vi "DSF.Engine.Execution.BuilderManager.Create.vi"(8 "error in (no error)":errorcluster, 10 "number of builders":i32, 11 "Framework Cache":refnum<class "DSF.Engine.Memory.Cache.Framework.lvclass">) -> (0 "error out":errorcluster, 3 "Builder Manager out":refnum<class "DSF.Engine.Execution.BuilderManager.lvclass">)   [LabVIEW 2016, in "DSF.Engine.lvlib" / "DSF.Engine.Execution.BuilderManager.lvclass"]
uses:
  DSF.Engine.Execution.BuilderManager.lvclass
  Cache/DSF.Engine.Memory.Cache.Framework.lvclass
  Builder/DSF.Engine.Execution.Builder.lvclass/DSF.Engine.Execution.Builder.ctl
  DSF.Engine.Execution.BuilderManager.lvclass/DSF.Engine.Execution.BuilderManager.ctl
  Builder/DSF.Engine.Execution.Builder.Set FIFOs.vi
  Builder/DSF.Engine.Execution.Builder.Set Status Pointers.vi
  Submodules/Memory/Source/Classes/Standard Types/Memory.Pointer.U32.New.vi
  Builder/DSF.Engine.Execution.Builder.Set Framework Cache.vi
  Submodules/Memory/Source/Classes/Standard Types/Memory.Pointer.U32.lvclass
  C:/Git/Sourcetree/DSF/Source/Submodules/Memory/Source/Classes/Internal/Memory.Pointer.Internal.lvclass
  Submodules/Memory/Source/Classes/Internal/Memory.Pointer.Internal.Allocate.vi
  Builder/DSF.Engine.Execution.Builder.lvclass
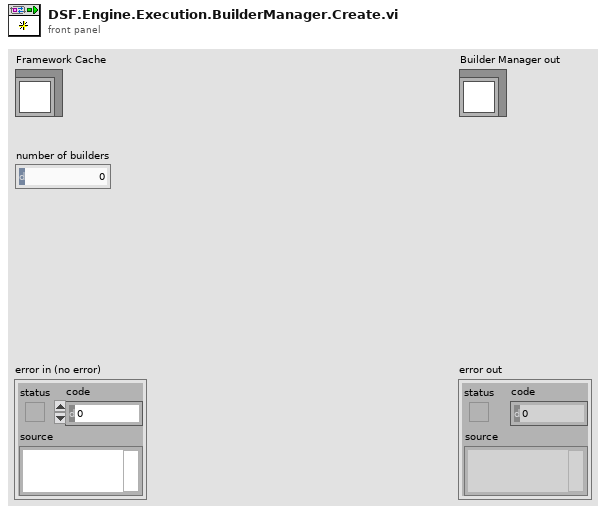
[diagram p1: front panel]
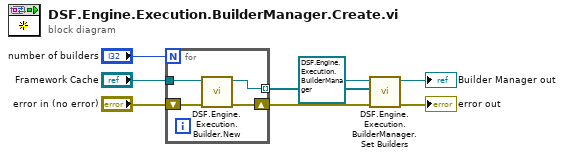
[diagram p0: block diagram]
diagram:
  n1 = for {
    N: "number of builders" -> [_]
    shift-right: [w11] -> w5
    shift-left: "error in (no error)" -> [w12]
    tunnel: [w10] -> w4 mode=indexing
    tunnel: "Framework Cache" -> [w9]
    n2 = call "DSF.Engine.Execution.Builder.New.vi"("error in (no error)"=w12, "Framework Cache"=w9) -> ("error out"=w11:errorcluster, "Builder"=w10:refnum<class "DSF.Engine.Execution.Builder.lvclass">)  [unwired: 8 in]
  }
  n3 = call "DSF.Engine.Execution.BuilderManager.Set Builders.vi"("error in (no error)"=w5, "Builders"=w4, "Builder Manager in"=refnum<class "DSF.Engine.Execution.BuilderManager.lvclass"> refnum) -> ("error out"=→"error out":errorcluster, "Builder Manager out"=→"Builder Manager out":refnum<class "DSF.Engine.Execution.BuilderManager.lvclass">)  [unwired: 7 in]
